vi "Request Update from Process.vi"(8 "error in (no error)":errorcluster, 11 "Ilde in":refnum<class "Idle.lvclass">) -> (0 "error out":errorcluster, 3 "Ilde out":refnum<class "Idle.lvclass">)   [LabVIEW 2012, in "Process States.lvlib" / "Idle.lvclass"]
doc: "Sends the Update message to the Process Actor."
uses:
  Idle.lvclass
  Process State/Process State.lvclass/Process State.ctl
  <vilib>/ActorFramework/Message Enqueuer/Message Enqueuer.lvclass/Message Enqueuer.ctl
  <vilib>/ActorFramework/Message Enqueuer/Enqueue.vi
  <vilib>/ActorFramework/Message Priority Queue/Priority Enqueue.vi
  Process Actor/Process Messages/Update Msg/Update Msg.lvclass
  Process State/Process State.lvclass
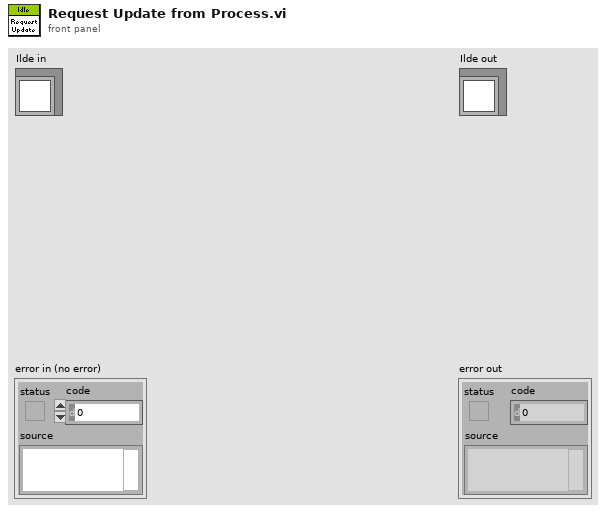
[diagram p1: front panel]
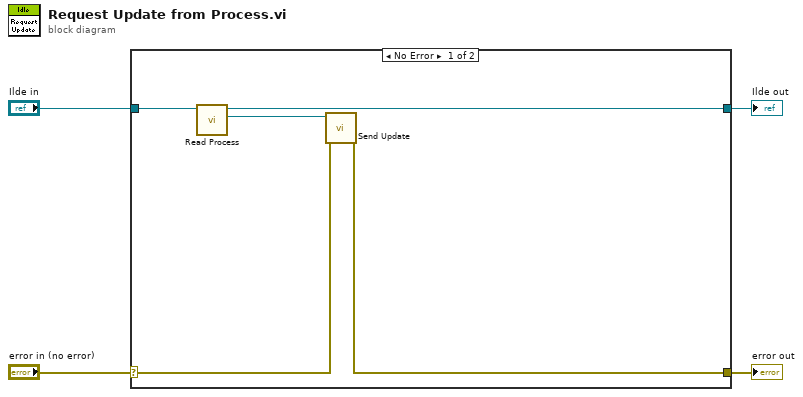
[diagram p0: block diagram]
diagram:
  n1 = case shown="No Error" "error in (no error)" {
    selector: "error in (no error)" -> [w6 w11]
    tunnel: [w5 w11] -> w3
    tunnel: [w8 w10] -> w1
    tunnel: "Ilde in" -> [w9 w10]
    frame No Error {
      n2 = call "Read Process.vi"("Process State in"=w9) -> ("Process Enqueuer"=w7:refnum<class "Message Enqueuer.lvclass">, "Process State out"=w8:refnum<class "Idle.lvclass">)  [unwired: 9 in]
      n3 = call "Send Update.vi"("error in (no error)"=w6, "Message Enqueuer"=w7) -> ("error out"=w5:errorcluster)  [unwired: 8 in, 1 out]
    }
    frame Error {
    }
  }
  "error out" <- w3
  "Ilde out" <- w1
